vi "start.vi"(8 "error in (no error)":errorcluster, 11 "PressureTransducerCompensator in":refnum<class "PressureTransducerCompensator.lvclass">) -> (0 "error out":errorcluster, 3 "PressureTransducerCompensator out":refnum<class "PressureTransducerCompensator.lvclass">)   [LabVIEW 2013, in "PressureTransducerCompensator.lvclass"]
uses:
  PressureTransducerCompensator.lvclass
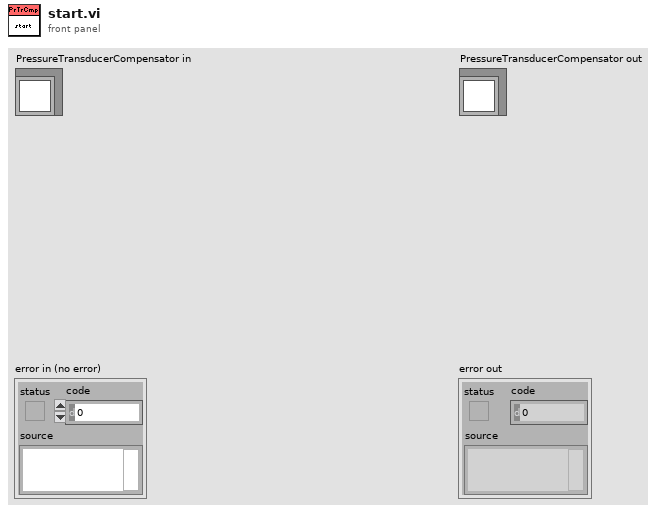
[diagram p1: front panel]
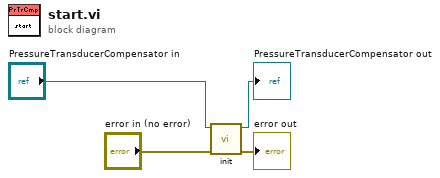
[diagram p0: block diagram]
diagram:
  n1 = call-dynamic "init.vi"("error in (no error)"="error in (no error)", "PressureTransducerCompensator in"="PressureTransducerCompensator in") -> ("error out"=→"error out":errorcluster, "PressureTransducerCompensator out"=→"PressureTransducerCompensator out":refnum<class "PressureTransducerCompensator.lvclass">)  [unwired: 8 in]
